vi "RunTest2.vi"(8 "error in (no error)":errorcluster, 11 "Prueba08 in":refnum<class "Prueba08.lvclass">) -> (0 "error out":errorcluster, 2 "resultado":string, 3 "Prueba08 out":refnum<class "Prueba08.lvclass">)   [LabVIEW 2019]
uses:
  <vilib>/Utility/miscctls.llb/LVRowAndColumnTypeDef.ctl
  Prueba/Prueba.lvclass
  Prueba08.lvclass
  Controles/EstadosP08.ctl
  MessageP08.ctl
  Prueba04/Control/Slide.ctl
  Prueba04/Prueba04.lvclass
  QMH/User Event - Stop/User Event - Stop.lvlib
  QMH/Message Queue/Message Queue.lvlib
  QMH/Message Queue/Enqueue Message (Single).vi
  ClusterGEN.ctl
  <vilib>/Utility/error.llb/DialogType.ctl
  <vilib>/Utility/error.llb/Error Cluster From Error Code.vi
  <vilib>/ErrorRing/Error Ring.xnode
  D:/REPO/GitHub/procal/Pruebas/Prueba/Prueba.lvclass
panel:
  out "data":string
  out "fila_tabla":i32
  out "ms":dbl
  out "ms":string[](array[string])
  out "max value":dbl
  out "tablaTipoPondTemp":string[](array[string])
  out "tablaNivelMaxRef":string[](array[string])
  out "Pict Ring 2":u16(ring)
  out "Pict Ring 3":u16(ring)
  out "cumple_no_cumple":bool
  out "Vref":dbl
  in  "Tab":enum32{"Page 1", "Page 2"}(tab)
  out "NivelRMSensayo":dbl=95.0
  out "frecuencia1":dbl=140.0
  out "rangoRef":string
  in  "guardar_Vref":bool
  in  "generar1":bool
  in  "AjusteAmp":T1=50.0 caption="Ajuste de amplitud [mV]" scale=0.0..5000.0
  out "voltaje1":dbl format="%.1f"
  out "frecuencia1":dbl format="%.1f"
  in  "seguir":bool
  in  "guardarParamLEQ":bool caption="PruebaSup"
  in  "Tm":i32=60 min=60
  in  "N":i32=1 min=1 max=9
  in  "TablaTempotal":string[][](table)
  in  "cb_ponderacionTemp":string(combo)="0"
  in  "genera2":bool caption="PruebaSup"
  in  "Tabla":string[][](table)
  in  "salir":bool
  out "cumple":bool
  out "no_cumple":bool
  out "voltaje2":dbl format="%#.1f"
  out "frecuencia2":dbl format="%#.1f"
  # "Elección Señal de Referencia\nsegún marca y modelo de sonómetro"
  # "Nivel RMS para Ensayo"
  # "Rango Referencia"
  # "Frecuencia"
  # "Monitoreo"
  # "Frecuencia"
  # "Hz"
  # "Voltaje"
  # "mV"
  # "8. Respuesta a trenes de ondas. IEC 61672-3: 2006 Cláusula 16"
  # "Tabla Resultados"
  # "Ingrese mediciones\naquí"
  # "Ingrese parámetros"
  # "Seleccione Tone Burst"
  # "N"
  # "Tm"
  # "Solo el máximo valor se \nregistrará en la tabla de Resultados"
  # "Cumple"
  # "No Cumple"
  # "8. Respuesta a trenes de ondas. IEC 61672-3: 2006 Cláusula 16"
  # "Monitoreo"
  # "Nivel RMS para Ensayo"
  # "dB"
  # "Voltaje"
  # "mV"
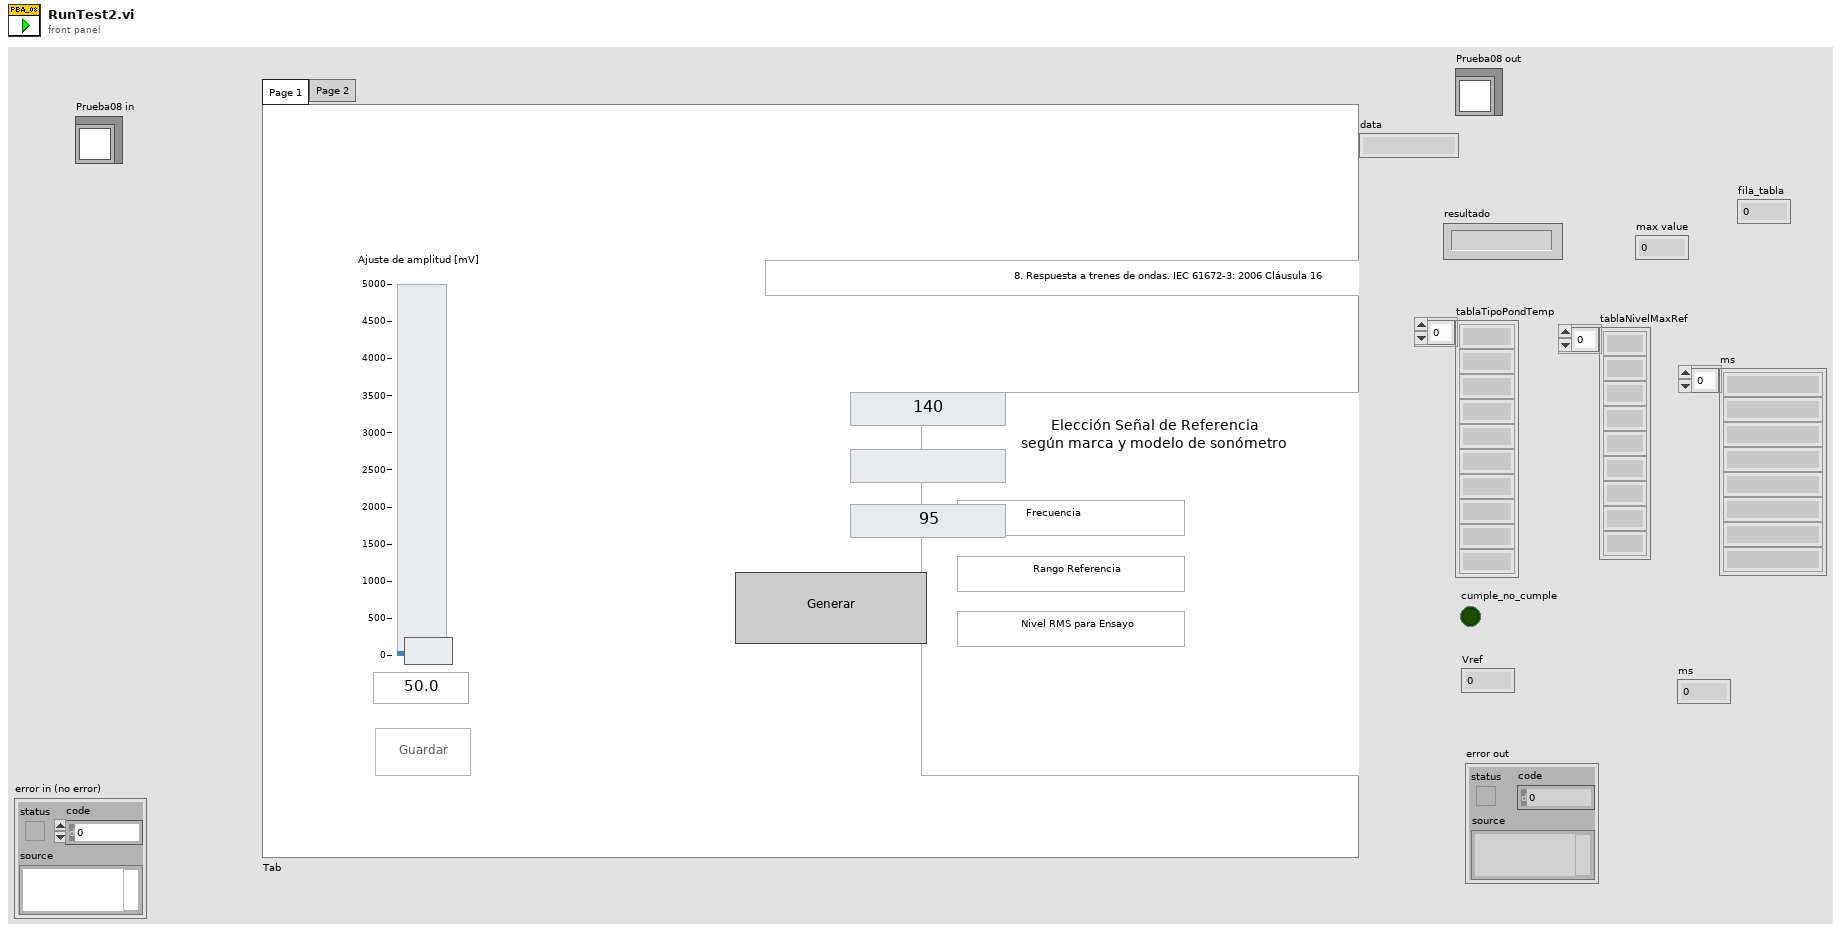
[diagram p1: front panel]
types:
  T1 = typedef "Prueba04.lvclass/Slide.ctl" = dbl
  T2 = typedef "LVRowAndColumnTypeDef.ctl" = cluster{"Row":i32, "Column":i32}
  T3 = typedef "Message Queue.lvlib/All Message Queues.ctl" = cluster{"MHL":refnum<queue>, "Inst_CNT90":refnum<queue>, "Inst_DS360":refnum<queue>, "Inst_Keithley2002":refnum<queue>, "Inst_DAQ":refnum<queue>, "BD":refnum<queue>, "Pistofono":refnum<queue>, "Nexus":refnum<queue>}
  T4 = enum32{"Page 1", "Page 2", "Page 3", "Page 4", "Page 5", "Page 6", "Page 7"}
  T5 = typedef "Prueba08.lvclass/ClusterGEN.ctl" = cluster{"frec":dbl, "amp":dbl, "ms_burst":dbl}
  T6 = enum8{"Enabled", "Disabled", "Disabled and Grayed Out"}
  T7 = cluster{"ControlName":string, "ControlReference":refnum<vi>}[]
  T8 = typedef "Prueba08.lvclass/MessageP08.ctl" = cluster{"Estados":T9, "Data":variant}
  T9 = typedef "Prueba08.lvclass/EstadosP08.ctl" = enum16{"Error", "DetieneInstrumentos", "InicializarInstrumentos", "inicio", "configuraTabla", "FrecAmp1", "FrecAmp2", "nivelMaxRef", "iniciarGEN", "iniciarGEN_burst", "detenerGEN", "llenaTablaTemporal", "guardaVref", "monitoreo", "ingresaMediciones", "guardaMediciones", "cumplimiento", "listo_evaluar", "evaluar", "LeerArchivoConfiguracion", "final", "salir"}
  T10 = typedef "DialogType.ctl" = u16
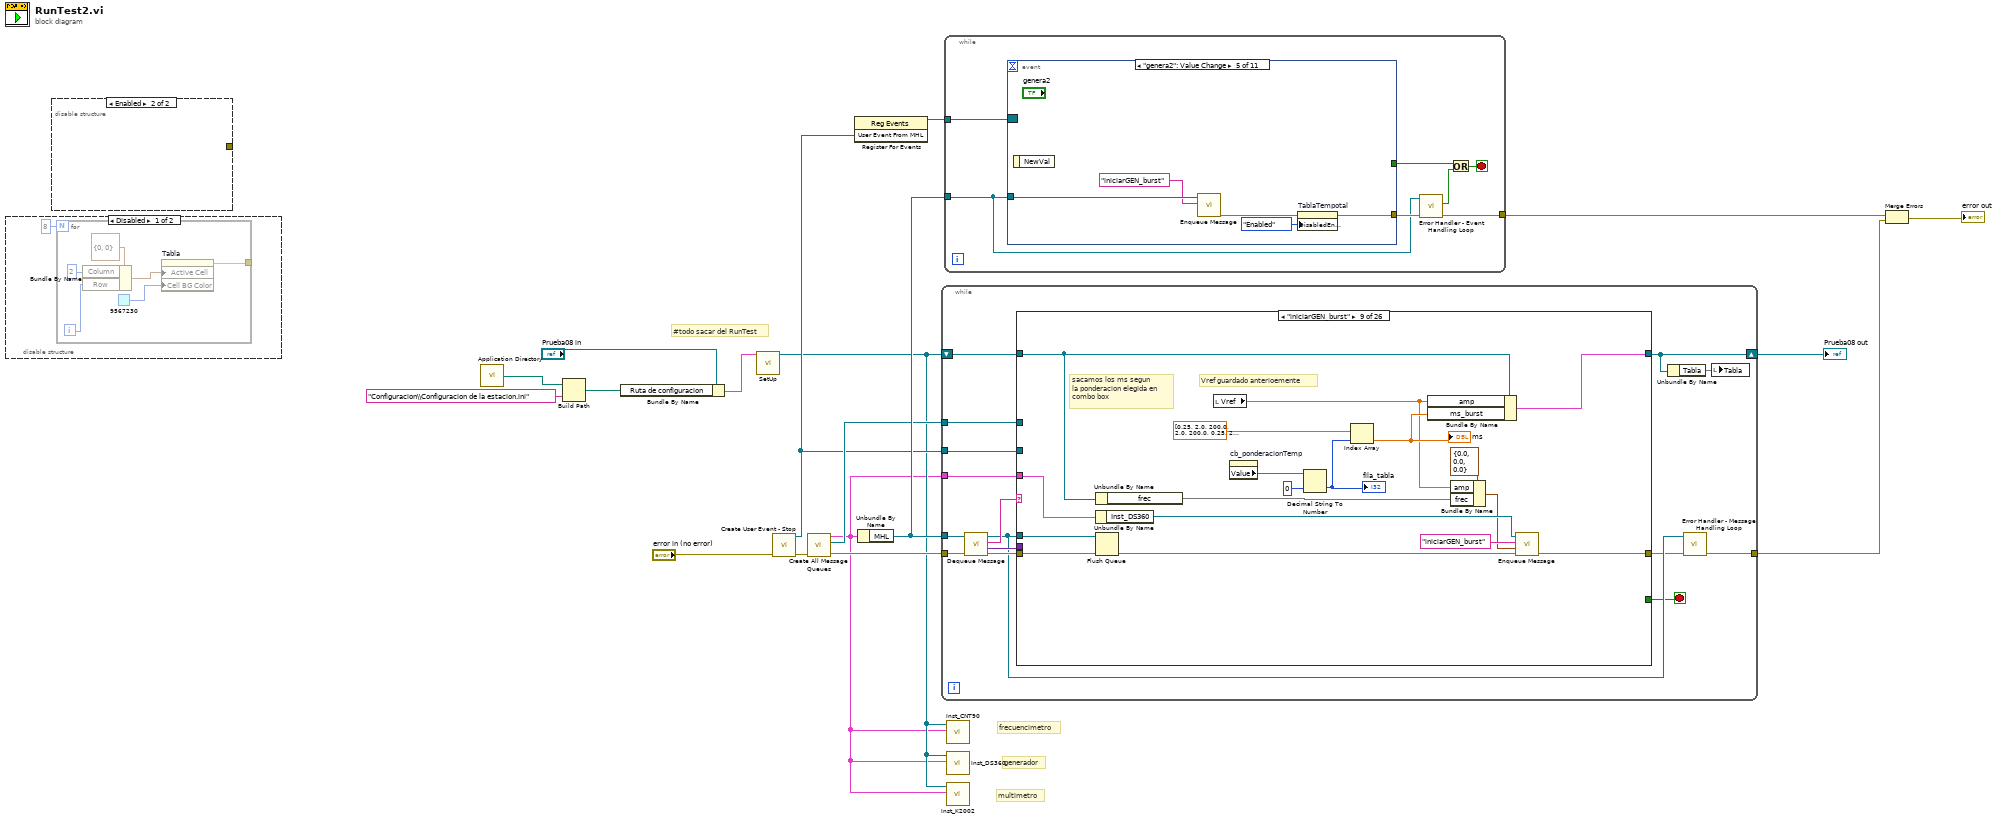
[diagram p0: block diagram]
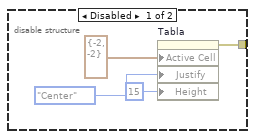
[diagram p3: hidden frame]
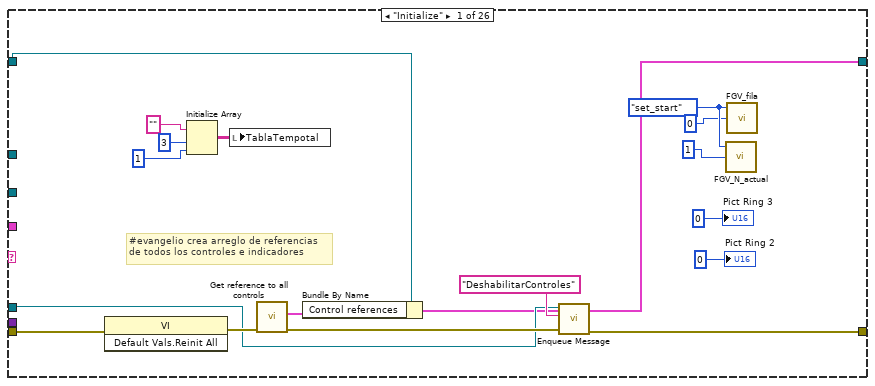
[diagram p4: hidden frame]
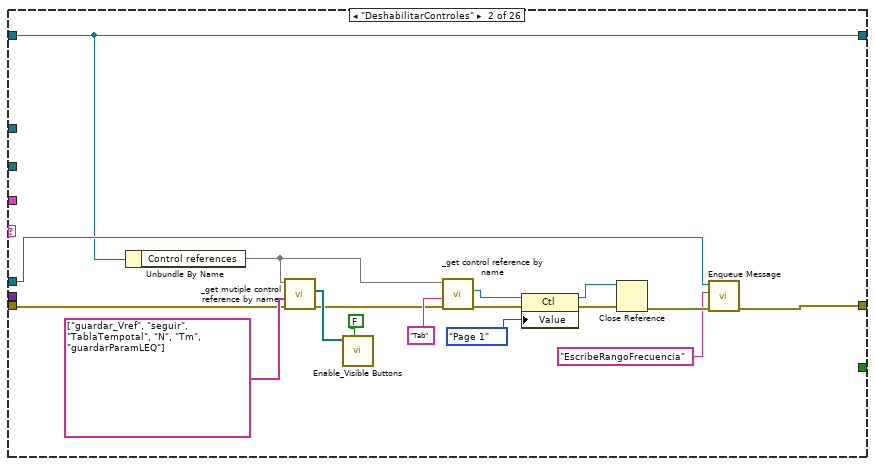
[diagram p5: hidden frame]
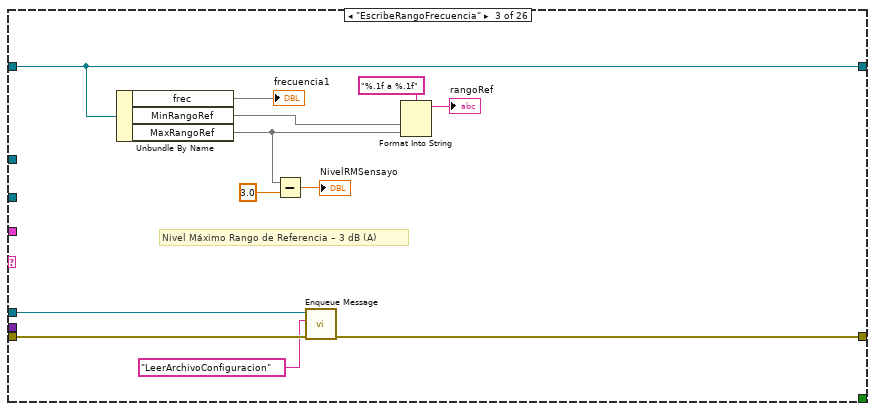
[diagram p6: hidden frame]
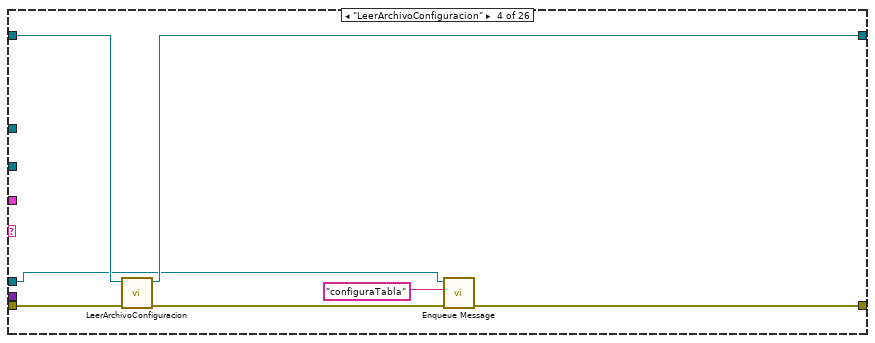
[diagram p7: hidden frame]
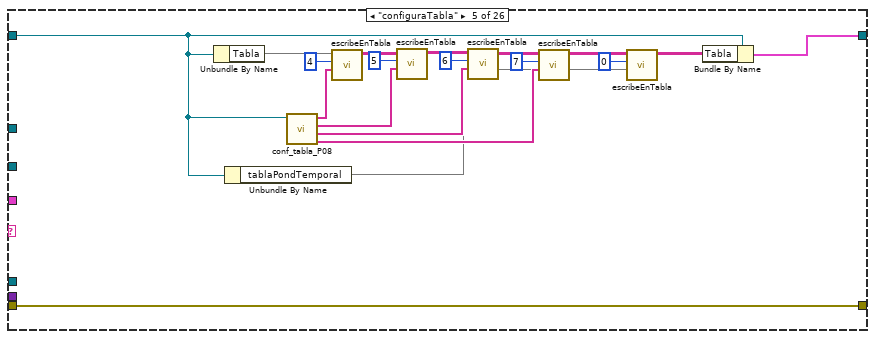
[diagram p8: hidden frame]
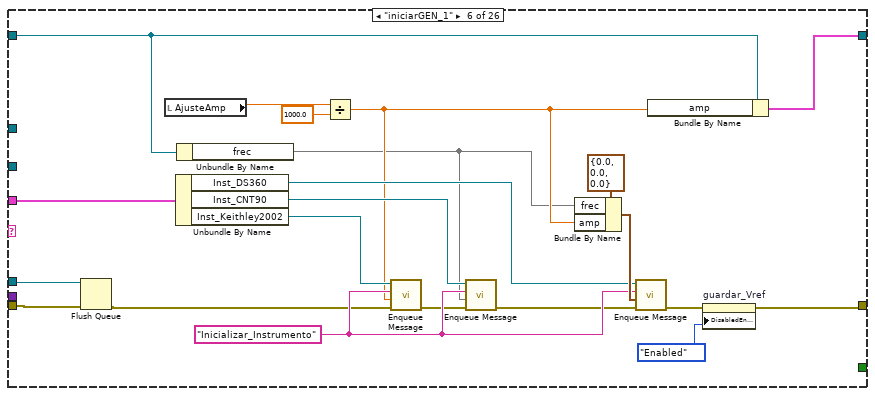
[diagram p9: hidden frame]
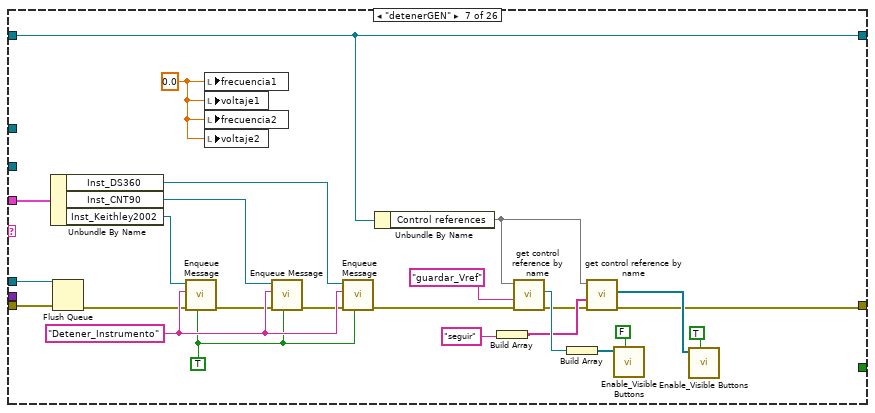
[diagram p10: hidden frame]
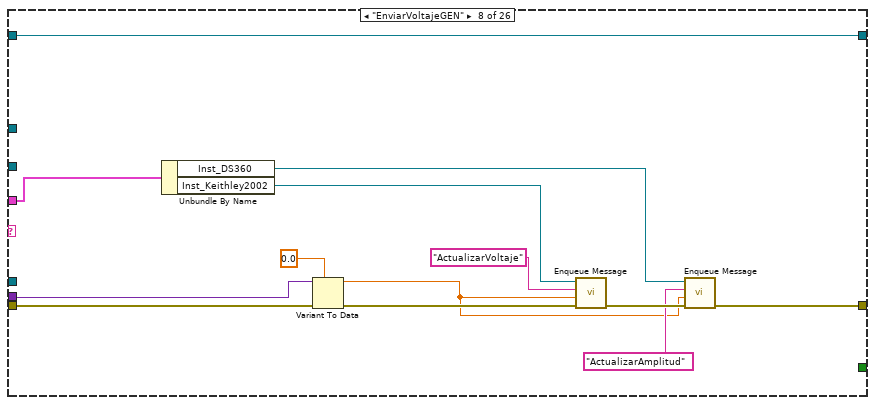
[diagram p11: hidden frame]
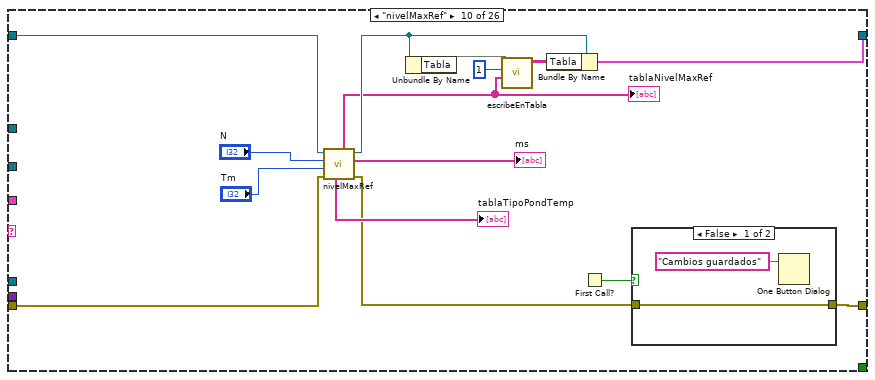
[diagram p12: hidden frame]
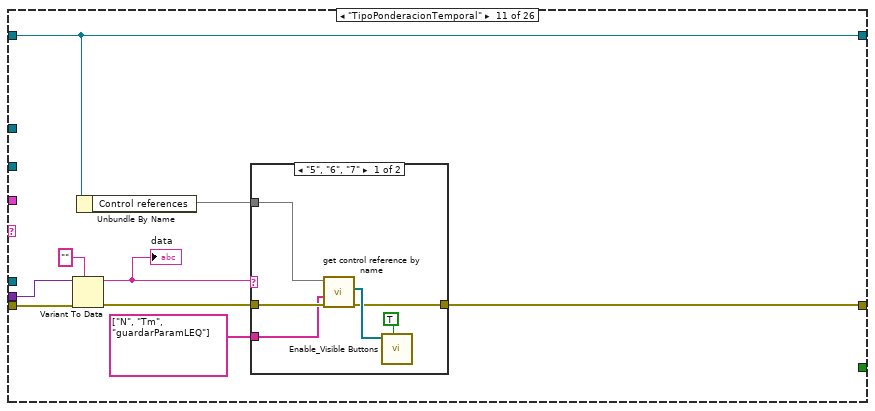
[diagram p14: hidden frame]
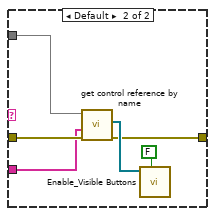
[diagram p15: hidden frame]
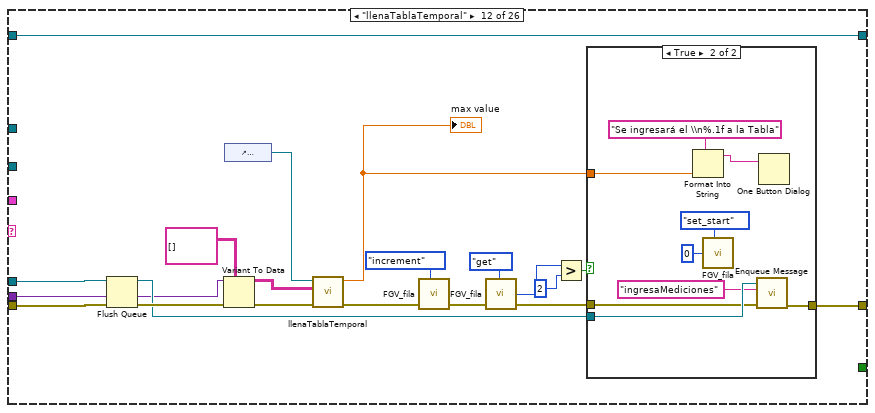
[diagram p16: hidden frame]
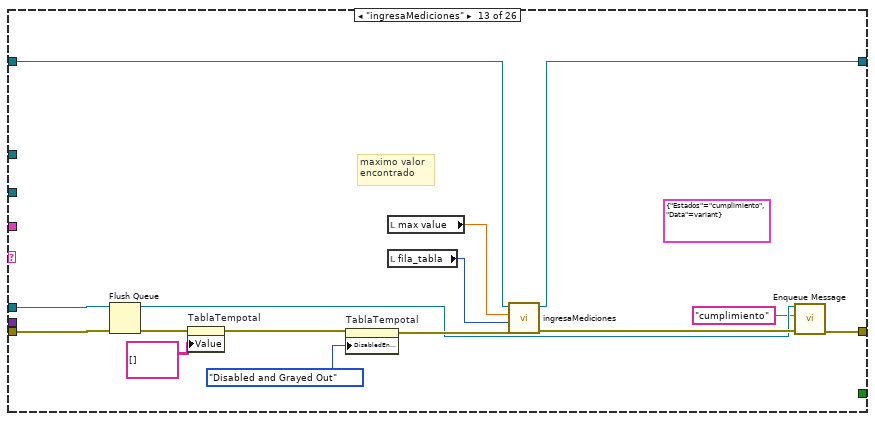
[diagram p18: hidden frame]
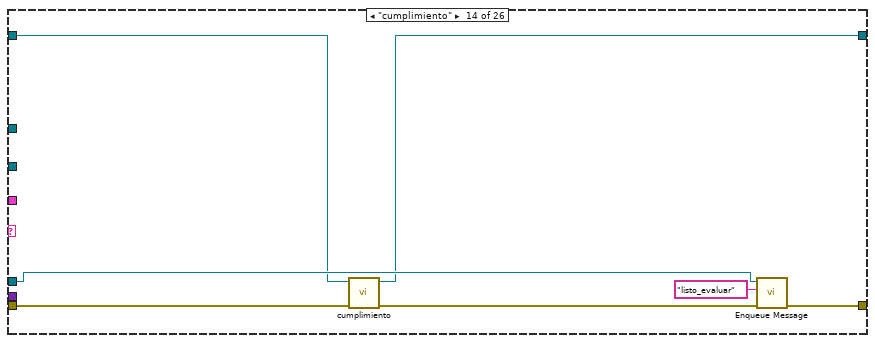
[diagram p19: hidden frame]
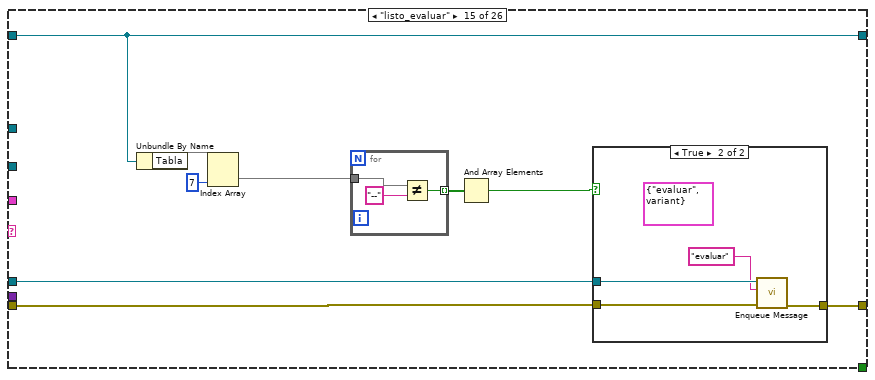
[diagram p20: hidden frame]
diagram:
  # "multimetro"
  # "generador"
  # "frecuencimetro"
  # "#todo sacar del RunTest"
  n1 = disable-structure shown="Disabled" {
    frame Disabled {
      n2 = for {
        N: 8 -> [_]
        tunnel: [w21] -> _
        i -> [w20]
        n3 = Bundle By Name(cluster=T2 {"Row"=0, "Column"=0} ("Active Cell:Active Cell"), "Column"=2, "Row"=w20) -> (w23:T2)
        n4 = property on="Tabla" class="Tbl (strict)"("Active Cell"=w23, "Cell BG Color"=u32 9567230) -> (error out=w21:errorcluster)  [unwired: 2 in, 1 out]
      }
    }
    frame Enabled {
    }
  }
  n5 = disable-structure shown="Enabled" {
    disable-tunnel: [w28 _] -> _
    frame Disabled {
      n6 = property on="Tabla" class="Tbl (strict)"("Active Cell"=T2 {"Row"=-2, "Column"=-2} ("Active Cell:Active Cell"), "Justify"=enum16{"Left", "Center", "Right"}."Center" ("Active Cell:Cell Justification"), "Height"=u32 15 ("Active Cell:Cell Font:Size")) -> (error out=w28:errorcluster)  [unwired: 2 in, 1 out]
    }
    frame Enabled {
    }
  }
  n7 = call <vilib>:"Application Directory.vi"() -> ("Application Directory"=w11:path)
  n8 = Build Path(base path=w11, name or relative path="Configuracion\\Configuracion de la estacion.ini") -> (appended path=w10:path)
  n9 = Bundle By Name(cluster="Prueba08 in", "Ruta de configuracion"=w10) -> (w13:cluster{})
  n10 = call-dynamic "SetUp.vi"("Prueba08 in"=w13) -> ("Prueba08 out"=w2:refnum<class "Prueba08.lvclass">)  [unwired: 9 in, 1 out]
  n11 = call "Create User Event - Stop.vi"("error in (no error)"="error in (no error)") -> ("error out"=w9:errorcluster, "User Event From MHL"=w4:refnum<user-event>)  [unwired: 9 in]
  n12 = call "Create All Message Queues.vi"("error in (no error)"=w9) -> ("error out"=w6:errorcluster, "PL Queues Array"=w5:refnum<queue>[], "All Message Queues out"=w1:T3)  [unwired: 8 in]
  n13 = register-events(w4) -> (reference out=w3:refnum<event-registration>)  [unwired: 2 in, 1 out]
  n14 = Unbundle By Name(w1) -> ("MHL"=w7:refnum<queue>)
  n15 = while {
    tunnel: w7 -> [w41]
    tunnel: w6 -> [w40]
    tunnel: [w34] -> w17
    shift-right: [w42] -> w15
    shift-left: w2 -> [w43]
    tunnel: w1 -> [w33]
    tunnel: w5 -> [w32]
    tunnel: w4 -> [w31]
    stop <- w30 stop-if-true
    n16 = call "Dequeue Message.vi"("error in (no error)"=w40, "Message Queue"=w41) -> ("error out"=w39:errorcluster, "Message Data"=w38:variant, "Message"=w37:string, "dup Message Queue"=w36:refnum<queue>)  [unwired: 6 in]
    n17 = case shown="\"iniciarGEN_burst\"" w37 {
      selector: w37 -> [_ _ _ _ _ _ _ _ _ _ _ _ _ _ _ _ _ _ _ _ _ _ w393 _ w420 _]
      tunnel: w38 -> [_ _ _ _ _ _ _ w164 _ _ w218 w244 _ _ _ _ _ _ w357 w368 _ w387 _ _ _ _]
      tunnel: w39 -> [w58 w66 w83 w98 w111 w125 w143 w165 w192 w206 w219 w251 w266 w283 w292 w308 w314 w321 w360 w371 w376 w388 w397 w408 _ w429]
      tunnel: [w56 w63 w80 w92 w111 w120 w141 w162 w177 w194 w212 w250 w267 w281 w291 w306 w314 w327 w354 w366 w376 w382 w390 w406 w419 w429] -> w35
      tunnel: w36 -> [w57 w65 w82 w94 _ w124 w142 _ w191 _ _ w248 w264 w280 w290 w307 _ w328 _ _ _ w381 w396 w407 _ _]
      tunnel: [w47 w64 w91 w97 w108 w138 w140 w174 w190 w201 w215 w245 w275 w279 w287 w304 w315 w330 w358 w369 w375 w389 w392 w413 w421 w430] -> w42
      tunnel: w43 -> [w48 w64 w91 w96 w100 w119 w140 w174 w176 w207 w215 w245 w276 w278 w287 w304 w315 w330 w359 w370 w375 w389 w392 w413 w421 w430]
      tunnel: w33 -> [_ _ _ _ _ w123 w144 w163 w184 _ _ _ _ _ _ _ _ _ _ _ _ _ _ _ _ _]
      tunnel: w32 -> [_ _ _ _ _ _ _ _ _ _ _ _ _ _ _ _ _ _ _ _ _ _ w395 _ _ _]
      tunnel: w31 -> [_ _ _ _ _ _ _ _ _ _ _ _ _ _ _ _ _ _ _ _ _ _ w394 _ _ _]
      tunnel: [_ _ _ _ _ _ _ _ _ _ _ _ _ _ _ _ _ _ _ _ _ _ w391 _ _ _] -> w30
      frame "Initialize" {
        w50 = enum16{"increment", "set_start", "get"}."set_start" ("action")
        # "#evangelio crea arreglo de referencias\nde todos los controles e indicadores"
        n18 = invoke class="VI" method="Default Vals.Reinit All"(error in=w58) -> (error out=w61:errorcluster)  [unwired: 2 in, 2 out]
        n19 = Initialize Array("", 3 ("dimension size"), 1 ("dimension size")) -> (w55:string[][])
        n20 = local write "TablaTempotal"(w55) -> ()
        n21 = call "Get reference to all controls.vi"("error in (no error)"=w61) -> ("error out"=w59:errorcluster, "Control references"=w60:T7)  [unwired: 5 in]
        n22 = Bundle By Name(cluster=w48, "Control references"=w60) -> (w47:cluster{})
        n23 = call-poly "Enqueue Message.vi"("error in (no error)"=w59, "Message"="DeshabilitarControles", "Message Queue"=w57) -> ("error out"=w56:errorcluster)  [unwired: 7 in, 1 out]
        n24 = call "FGV_N_actual.vi"("N_actual in"=1 ("fila_inicial"), "action"=w50) -> ()  [unwired: 2 in, 2 out]
        n25 = call "FGV_fila.vi"("fila_inicial"=0, "action"=w50) -> ()  [unwired: 2 in, 2 out]
        "Pict Ring 2" <- u16 0 ("Pict Ring 2")
        "Pict Ring 3" <- u16 0 ("Pict Ring 3")
      }
      frame "DeshabilitarControles" {
        n26 = Unbundle By Name(w64) -> ("Control references"=w75)
        n27 = call "_get mutiple control reference by name.vi"("error in (no error)"=w66, "Control names"=string[] ["guardar_Vref", "seguir", "TablaTempotal", "N", "Tm", "guardarParamLEQ"], "Control references"=w75) -> ("error out"=w72:errorcluster, "References"=w73:refnum<vi>[])  [unwired: 3 in]
        n28 = call "Enable_Visible Buttons.vi"("Enable? (T)"=FALSE, "Controls Ref Array"=w73) -> ()  [unwired: 10 in]
        n29 = call "_get control reference by name.vi"("error in (no error)"=w72, "Control name"="Tab" ("Message"), "Control references"=w75) -> ("error out"=w79:errorcluster, "Ctl Refnum"=w77:refnum<vi>)  [unwired: 3 in]
        n30 = property class="Ctl"(reference=w77, error in=w79, "Value"=T4."Page 1" ("Tab_Prueba04")) -> (reference out=w68:refnum<vi>, error out=w70:errorcluster)
        n31 = Close Reference(reference=w68, error in (no error)=w70) -> (error out=w69:errorcluster)
        n32 = call-poly "Enqueue Message.vi"("error in (no error)"=w69, "Message"="EscribeRangoFrecuencia", "Message Queue"=w65) -> ("error out"=w63:errorcluster)  [unwired: 7 in, 1 out]
      }
      frame "EscribeRangoFrecuencia" {
        # "Nivel Máximo Rango de Referencia – 3 dB (A)"
        n33 = Unbundle By Name(w91) -> ("frec"=→"frecuencia1", "MinRangoRef"=w87, "MaxRangoRef"=w86)
        n34 = Subtract(x=w86, y=3.0) -> (x-y=→"NivelRMSensayo":dbl)
        n35 = call-poly "Enqueue Message.vi"("error in (no error)"=w83, "Message"="LeerArchivoConfiguracion", "Message Queue"=w82) -> ("error out"=w80:errorcluster)  [unwired: 7 in, 1 out]
        n36 = Format Into String(format string="%.1f a %.1f", w87, w86) -> (resulting string=→"rangoRef":string)  [unwired: 2 in, 1 out]
      }
      frame "LeerArchivoConfiguracion" {
        n37 = call "LeerArchivoConfiguracion.vi"("error in"=w98, "Prueba31 in"=w96) -> ("error out"=w95:errorcluster, "Prueba31 out"=w97:refnum<class "Prueba08.lvclass">)  [unwired: 8 in]
        n38 = call-poly "Enqueue Message.vi"("error in (no error)"=w95, "Message"="configuraTabla", "Message Queue"=w94) -> ("error out"=w92:errorcluster)  [unwired: 7 in, 1 out]
      }
      frame "configuraTabla" {
        n39 = Unbundle By Name(w100) -> ("Tabla"=w107)
        n40 = Unbundle By Name(w100) -> ("tablaPondTemporal"=w99)
        n41 = call "conf_tabla_P08.vi"("Prueba07 out"=w100) -> ("cumplimiento"=w103:string[], "Tol -"=w104:string[], "Tol +"=w105:string[], "incertidumbre"=w106:string[])  [unwired: 7 in]
        n42 = call "escribeEnTabla.vi"("parametros"=w106, "col"=4, "tabla in"=w107) -> ("tabla out"=w117:string[][])  [unwired: 8 in]
        n43 = call "escribeEnTabla.vi"("parametros"=w105, "col"=5, "tabla in"=w117) -> ("tabla out"=w116:string[][])  [unwired: 8 in]
        n44 = call "escribeEnTabla.vi"("parametros"=w104, "col"=6, "tabla in"=w116) -> ("tabla out"=w112:string[][])  [unwired: 8 in]
        n45 = call "escribeEnTabla.vi"("parametros"=w103, "col"=7, "tabla in"=w112) -> ("tabla out"=w110:string[][])  [unwired: 8 in]
        n46 = call "escribeEnTabla.vi"("parametros"=w99, "col"=0, "tabla in"=w110) -> ("tabla out"=w102:string[][])  [unwired: 8 in]
        n47 = Bundle By Name(cluster=w100, "Tabla"=w102) -> (w108:cluster{})
      }
      frame "iniciarGEN_1" {
        w133 = "Inicializar_Instrumento" ("Message")
        n48 = Flush Queue(queue=w124, error in (no error)=w125) -> (error out=w127:errorcluster)  [unwired: 2 out]
        n49 = local read "AjusteAmp"() -> (w137:T1)
        n50 = Unbundle By Name(w123) -> ("Inst_DS360"=w128:refnum<queue>, "Inst_CNT90"=w126:refnum<queue>, "Inst_Keithley2002"=w135:refnum<queue>)
        n51 = Unbundle By Name(w119) -> ("frec"=w118)
        n52 = Divide(x=w137, y=T1 1000.0) -> (x/y=w121:T1)
        n53 = call-poly "Enqueue Message.vi"("error in (no error)"=w127, "Message Data"=w121, "Message"=w133, "Message Queue"=w135) -> ("error out"=w132:errorcluster)  [unwired: 6 in, 1 out]
        n54 = call-poly "Enqueue Message.vi"("error in (no error)"=w132, "Message Data"=w118, "Message"=w133, "Message Queue"=w126) -> ("error out"=w131:errorcluster)  [unwired: 6 in, 1 out]
        n55 = Bundle By Name(cluster=T5 {"frec"=0.0, "amp"=0.0, "ms_burst"=0.0} ("clusterGEN"), "frec"=w118, "amp"=w121) -> (w134:T5)
        n56 = call-poly "Enqueue Message.vi"("error in (no error)"=w131, "Message Data"=w134, "Message"=w133, "Message Queue"=w128) -> ("error out"=w129:errorcluster)  [unwired: 6 in, 1 out]
        n57 = Bundle By Name(cluster=w119, "amp"=w121) -> (w138:cluster{})
        n58 = property on="guardar_Vref" class="Bool"(error in=w129, "DisabledEnum"=T6."Enabled" ("Disabled")) -> (error out=w120:errorcluster)  [unwired: 1 in, 1 out]
      }
      frame "detenerGEN" {
        w139 = 0.0 ("frecuencia1")
        w157 = TRUE ("Priority Message? (F)")
        w158 = "Detener_Instrumento"
        n59 = Unbundle By Name(w144) -> ("Inst_DS360"=w159:refnum<queue>, "Inst_CNT90"=w160:refnum<queue>, "Inst_Keithley2002"=w161:refnum<queue>)
        n60 = Flush Queue(queue=w142, error in (no error)=w143) -> (error out=w146:errorcluster)  [unwired: 2 out]
        n61 = call-poly "Enqueue Message.vi"("Priority Message? (F)"=w157, "Message"=w158, "Message Queue"=w161) -> ()  [unwired: 7 in, 2 out]
        n62 = local write "frecuencia1"(w139) -> ()
        n63 = local write "voltaje1"(w139) -> ()
        n64 = local write "frecuencia2"(w139) -> ()
        n65 = local write "voltaje2"(w139) -> ()
        n66 = call-poly "Enqueue Message.vi"("Priority Message? (F)"=w157, "Message"=w158, "Message Queue"=w160) -> ()  [unwired: 7 in, 2 out]
        n67 = call-poly "Enqueue Message.vi"("Priority Message? (F)"=w157, "error in (no error)"=w146, "Message"=w158, "Message Queue"=w159) -> ("error out"=w155:errorcluster)  [unwired: 6 in, 1 out]
        n68 = Unbundle By Name(w140) -> ("Control references"=w150)
        n69 = Build Array("seguir" ("String")) -> (w147:string[])
        n70 = call-poly "get control reference by name.vi"("error in (no error)"=w155, "Control name"="guardar_Vref" ("String"), "Control references"=w150) -> ("error out"=w145:errorcluster, "Ctl Refnum"=w153:refnum<vi>)  [unwired: 3 in]
        n71 = Build Array(w153) -> (w152:refnum<vi>[])
        n72 = call-poly "get control reference by name.vi"("error in (no error)"=w145, "Control names"=w147, "Control references"=w150) -> ("error out"=w141:errorcluster, "References"=w149:refnum<vi>[])  [unwired: 3 in]
        n73 = call "Enable_Visible Buttons.vi"("Enable? (T)"=FALSE, "Controls Ref Array"=w152) -> ()  [unwired: 10 in]
        n74 = call "Enable_Visible Buttons.vi"("Enable? (T)"=TRUE, "Controls Ref Array"=w149) -> ()  [unwired: 10 in]
      }
      frame "EnviarVoltajeGEN" {
        n75 = Unbundle By Name(w163) -> ("Inst_DS360"=w168:refnum<queue>, "Inst_Keithley2002"=w173:refnum<queue>)
        n76 = Variant To Data(error in=w165, type=0.0, Variant=w164) -> (data=w166:dbl, error out=w171:errorcluster)
        n77 = call-poly "Enqueue Message.vi"("error in (no error)"=w171, "Message Data"=w166, "Message"="ActualizarVoltaje", "Message Queue"=w173) -> ("error out"=w169:errorcluster)  [unwired: 6 in, 1 out]
        n78 = call-poly "Enqueue Message.vi"("error in (no error)"=w169, "Message Data"=w166, "Message"="ActualizarAmplitud", "Message Queue"=w168) -> ("error out"=w162:errorcluster)  [unwired: 6 in, 1 out]
      }
      frame "iniciarGEN_burst" {
        # "sacamos los ms segun\nla ponderacion elegida en\ncombo box"
        # "Vref guardado anterioemente"
        n79 = Unbundle By Name(w184) -> ("Inst_DS360"=w182:refnum<queue>)
        n80 = Flush Queue(queue=w191, error in (no error)=w192) -> (error out=w183:errorcluster)  [unwired: 2 out]
        n81 = Unbundle By Name(w176) -> ("frec"=w175)
        n82 = local read "Vref"() -> (w178:dbl)
        n83 = property on="cb_ponderacionTemp" class="CmbBox"() -> ("Value"=w187:string)  [unwired: 2 in, 2 out]
        n84 = Decimal String To Number(string=w187, default (0L)=0 ("default (0 I32)")) -> (number=w185:i32)  [unwired: 1 in, 1 out]
        "fila_tabla" <- w185
        n85 = Index Array(array=dbl[] [0.25, 2.0, 200.0, 2.0, 200.0, 0.25, 2.0, 200.0], index=w185) -> (element=w188:dbl)
        "ms" <- w188
        n86 = Bundle By Name(cluster=w176, "amp"=w178, "ms_burst"=w188) -> (w190:cluster{})
        n87 = Bundle By Name(cluster=T5 {"frec"=0.0, "amp"=0.0, "ms_burst"=0.0} ("clusterGEN"), "amp"=w178, "frec"=w175) -> (w179:T5)
        n88 = call-poly "Enqueue Message.vi"("error in (no error)"=w183, "Message Data"=w179, "Message"="iniciarGEN_burst", "Message Queue"=w182) -> ("error out"=w177:errorcluster)  [unwired: 6 in, 1 out]
      }
      frame "nivelMaxRef" {
        n89 = call "nivelMaxRef.vi"("error in (no error)"=w206, "Tm"="Tm", "N"="N", "Prueba08 in"=w207) -> ("error out"=w195:errorcluster, "ms"=→"ms":string[], "Prueba08 out"=w205:refnum<class "Prueba08.lvclass">, "tablaNivelMaxRef"=w202:string[], "tablaTipoPondTemp"=→"tablaTipoPondTemp":string[])  [unwired: 2 in, 1 out]
        "tablaNivelMaxRef" <- w202
        n90 = Unbundle By Name(w205) -> ("Tabla"=w204)
        n91 = call "escribeEnTabla.vi"("parametros"=w202, "col"=1, "tabla in"=w204) -> ("tabla out"=w200:string[][])  [unwired: 8 in]
        n92 = Bundle By Name(cluster=w205, "Tabla"=w200) -> (w201:cluster{})
        n93 = First Call?() -> (First Call?: T/F=w193:bool)
        n94 = case shown="False" w193 {
          tunnel: w195 -> [w208 w210]
          tunnel: [w208 w210] -> w194
          frame False {
            n95 = One Button Dialog(message="Cambios guardados") -> ()  [unwired: 1 in, 1 out]
          }
          frame True {
          }
        }
      }
      frame "TipoPonderacionTemporal" {
        n96 = Variant To Data(error in=w219, type="", Variant=w218) -> (data=w216:string, error out=w213:errorcluster)
        "data" <- w216
        n97 = Unbundle By Name(w215) -> ("Control references"=w214)
        n98 = case shown="\"5\", \"6\", \"7\"" w216 {
          tunnel: w214 -> [w222 w228]
          tunnel: w213 -> [w221 w227]
          tunnel: [w223 w229] -> w212
          tunnel: string[] ["N", "Tm", "guardarParamLEQ"] ("String") -> [w220 w226]
          frame "5", "6", "7" {
            n99 = call-poly "get control reference by name.vi"("error in (no error)"=w221, "Control names"=w220, "Control references"=w222) -> ("error out"=w223:errorcluster, "References"=w224:refnum<vi>[])  [unwired: 3 in]
            n100 = call "Enable_Visible Buttons.vi"("Enable? (T)"=TRUE, "Controls Ref Array"=w224) -> ()  [unwired: 10 in]
          }
          frame Default {
            n101 = call-poly "get control reference by name.vi"("error in (no error)"=w227, "Control names"=w226, "Control references"=w228) -> ("error out"=w229:errorcluster, "References"=w230:refnum<vi>[])  [unwired: 3 in]
            n102 = call "Enable_Visible Buttons.vi"("Enable? (T)"=FALSE, "Controls Ref Array"=w230) -> ()  [unwired: 10 in]
          }
        }
      }
      frame "llenaTablaTemporal" {
        n103 = Flush Queue(queue=w248, error in (no error)=w251) -> (queue out=w247:refnum<queue>, error out=w249:errorcluster)  [unwired: 1 out]
        n104 = Variant To Data(error in=w249, type=string[][] [] ("NewVal"), Variant=w244) -> (data=w242:string[][], error out=w241:errorcluster)
        n105 = control-ref of="TablaTempotal"() -> (w243:refnum<vi>)
        n106 = call "llenaTablaTemporal.vi"("Tbl Refnum"=w243, "New Value"=w242, "error out"=w241) -> ("max value"=w232:dbl, "error in (no error)"=w240:errorcluster)  [unwired: 6 in]
        "max value" <- w232
        n107 = call "FGV_fila.vi"("error in (no error)"=w240, "action"=enum16{"increment", "set_start", "get"}."increment") -> ("error out"=w239:errorcluster)  [unwired: 2 in, 1 out]
        n108 = call "FGV_fila.vi"("error in (no error)"=w239, "action"=enum16{"increment", "set_start", "get"}."get") -> ("error out"=w237:errorcluster, "fila out"=w235:i32)  [unwired: 2 in]
        n109 = Greater?(x=w235, y=2) -> (0:w233:bool)
        n110 = case shown="True" w233 {
          tunnel: [w252 w261] -> w250
          tunnel: w247 -> [_ w260]
          tunnel: w237 -> [w252 w259]
          tunnel: w232 -> [_ w255]
          frame False {
          }
          frame True {
            n111 = Format Into String(format string="Se ingresará el \\n%.1f a la Tabla" ("message"), w255) -> (resulting string=w254:string)  [unwired: 2 in, 1 out]
            n112 = call "FGV_fila.vi"("fila_inicial"=0, "action"=enum16{"increment", "set_start", "get"}."set_start") -> ()  [unwired: 2 in, 2 out]
            n113 = call-poly "Enqueue Message.vi"("error in (no error)"=w259, "Message"="ingresaMediciones", "Message Queue"=w260) -> ("error out"=w261:errorcluster)  [unwired: 7 in, 1 out]
            n114 = One Button Dialog(message=w254) -> ()  [unwired: 1 in, 1 out]
          }
        }
      }
      frame "ingresaMediciones" {
        (unwired) T8 {"Estados"=enum."cumplimiento", "Data"=variant} ("element")
        # "maximo valor\nencontrado"
        n115 = Flush Queue(queue=w264, error in (no error)=w266) -> (queue out=w263:refnum<queue>, error out=w265:errorcluster)  [unwired: 1 out]
        n116 = property on="TablaTempotal" class="Tbl (strict)"(error in=w265, "Value"=string[][] [] ("TablaTempotal")) -> (error out=w271:errorcluster)  [unwired: 1 in, 1 out]
        n117 = property on="TablaTempotal" class="Tbl (strict)"(error in=w271, "DisabledEnum"=T6."Disabled and Grayed Out" ("Disabled")) -> (error out=w270:errorcluster)  [unwired: 1 in, 1 out]
        n118 = local read "max value"() -> (w274:dbl)
        n119 = local read "fila_tabla"() -> (w273:i32)
        n120 = call "ingresaMediciones.vi"("error in (no error)"=w270, "fila tabla"=w273, "max value"=w274, "Prueba08 in"=w276) -> ("error out"=w268:errorcluster, "Prueba08 out"=w275:refnum<class "Prueba08.lvclass">)  [unwired: 6 in]
        n121 = call-poly "Enqueue Message.vi"("error in (no error)"=w268, "Message"="cumplimiento", "Message Queue"=w263) -> ("error out"=w267:errorcluster)  [unwired: 7 in, 1 out]
      }
      frame "cumplimiento" {
        n122 = call "cumplimiento.vi"("error in (no error)"=w283, "Prueba08 in"=w278) -> ("error out"=w282:errorcluster, "Prueba08 out"=w279:refnum<class "Prueba08.lvclass">)  [unwired: 8 in]
        n123 = call-poly "Enqueue Message.vi"("error in (no error)"=w282, "Message"="listo_evaluar", "Message Queue"=w280) -> ("error out"=w281:errorcluster)  [unwired: 7 in, 1 out]
      }
      frame "listo_evaluar" {
        n124 = Unbundle By Name(w287) -> ("Tabla"=w286)
        n125 = Index Array(array=w286, index (col)=7 ("disabled index (col)")) -> (element=w285)  [unwired: 1 in]
        n126 = for {
          tunnel: [w300] -> w288 mode=indexing
          tunnel: w285 -> [w298]
          n127 = Not Equal?(x=w298, y="--") -> (x != y?=w300:bool)
        }
        n128 = And Array Elements(Boolean array=w288) -> (logical AND=w284:bool)
        n129 = case shown="True" w284 {
          tunnel: w292 -> [w293 w297]
          tunnel: [w293 w296] -> w291
          tunnel: w290 -> [_ w295]
          frame False {
          }
          frame True {
            (unwired) T8 {"Estados"=enum."evaluar", "Data"=variant} ("MessageP08")
            n130 = call-poly "Enqueue Message.vi"("error in (no error)"=w297, "Message"="evaluar", "Message Queue"=w295) -> ("error out"=w296:errorcluster)  [unwired: 7 in, 1 out]
          }
        }
      }
      frame "evaluar" {
        # "si todos cumplen\nentonces el ensayo\ncumple"
        n131 = Unbundle By Name(w304) -> ("Tabla"=w303)
        n132 = call-poly "Enqueue Message.vi"("error in (no error)"=w308, "Message"="final", "Message Queue"=w307) -> ("error out"=w306:errorcluster)  [unwired: 7 in, 1 out]
        n133 = Index Array(array=w303, index (col)=7 ("disabled index (col)")) -> (element=w302)  [unwired: 1 in]
        n134 = for {
          tunnel: [w313] -> w310 mode=indexing
          tunnel: w302 -> [w311]
          n135 = Equal?(x=w311, y="Cumple") -> (x = y?=w313:bool)
        }
        n136 = And Array Elements(Boolean array=w310) -> (logical AND=→"cumple_no_cumple":bool)
      }
      frame "final" {
        n137 = local read "cumple_no_cumple"() -> (w316:bool)
        "cumple" <- w316
        n138 = Not(x=w316) -> (.not. x?=→"no_cumple":bool)
        n139 = Select(t="Cumple", s=w316, f="No Cumple") -> (s? t:f=→"resultado":string)
      }
      frame "iniciarGEN_burst_2" {
        n140 = property on="cb_ponderacionTemp" class="CmbBox"(error in=w321) -> ("Value"=w324:string)  [unwired: 1 in, 2 out]
        n141 = local read "N"() -> (w326:i32)
        n142 = local read "Tm"() -> (w329:i32)
        n143 = case shown="\"5\"..\"7\"" w324 {
          tunnel: w321 -> [w334 w345]
          tunnel: w329 -> [w333 w344]
          tunnel: w326 -> [_ w343]
          tunnel: [w332 w340] -> w323
          tunnel: [2 ("N_actual out") w339] -> w322
          frame "0".."4", Default {
            n144 = disable-structure shown="Disabled" {
              disable-tunnel: w334 -> [w337 w338]
              disable-tunnel: w333 -> [w336 _]
              disable-tunnel: [w335 w338] -> w332
              frame Disabled {
                n145 = call "estadoToneBurst_FastSlow.vi"("error in (no error)"=w337, "Tm"=w336) -> ("error out"=w335:errorcluster)  [unwired: 9 in]
              }
              frame Enabled {
              }
            }
          }
          frame "5".."7" {
            n146 = call "estadoToneBurst.vi"("error in (no error)"=w345, "Tm"=w344, "N"=w343) -> ("error out"=w341:errorcluster)  [unwired: 7 in, 1 out]
            n147 = call "FGV_N_actual.vi"("error in (no error)"=w341, "action"=enum16{"increment", "set_start", "get"}."increment") -> ("error out"=w340:errorcluster, "N_actual out"=w339:i32)  [unwired: 2 in]
          }
        }
        n148 = Greater?(x=w322, y=w326) -> (0:w325:bool)
        n149 = case shown="True" w325 {
          tunnel: w328 -> [w349 _]
          tunnel: [w348 w353] -> w327
          tunnel: w323 -> [w347 w353]
          frame False {
            n150 = call-poly "Enqueue Message.vi"("error in (no error)"=w347, "Message"="iniciarGEN_burst", "Message Queue"=w349) -> ("error out"=w348:errorcluster)  [unwired: 7 in, 1 out]
          }
          frame True {
            n151 = One Button Dialog(message="Ingrese las mediciones \nen la Tabla Temporal") -> ()  [unwired: 1 in, 1 out]
            n152 = call "FGV_N_actual.vi"("N_actual in"=1, "action"=enum16{"increment", "set_start", "get"}."set_start") -> ()  [unwired: 2 in, 2 out]
          }
        }
      }
      frame "DatoRecibidoCNT90" {
        n153 = Variant To Data(error in=w360, type=0.0 ("y"), Variant=w357) -> (data=w355:dbl, error out=w354:errorcluster)
        "frecuencia2" <- w355
        "frecuencia1" <- w355
        n154 = Bundle By Name(cluster=w359, "frecMedida"=w355) -> (w358:cluster{})
      }
      frame "DatoRecibidoK2002" {
        n155 = Variant To Data(error in=w371, type=0.0 ("y"), Variant=w368) -> (data=w362:dbl, error out=w366:errorcluster)
        n156 = Multiply(x=w362, y=1000.0) -> (x*y=w361:dbl)
        "voltaje2" <- w361
        n157 = Multiply(x=w362, y=1000.0) -> (x*y=→"voltaje1":dbl)
        n158 = Bundle By Name(cluster=w370, "voltMedido"=w361) -> (w369:cluster{})
      }
      frame "guardaVref" {
        n159 = local read "AjusteAmp"() -> (w374:T1)
        n160 = Divide(x=w374, y=T1 1000.0) -> (x/y=w372:T1)
        "Vref" <- w372
        n161 = Number To Fractional String(number=w372, precision (6)=i16 3) -> (F-format string=w377:string)  [unwired: 2 in]
        n162 = Format Into String(format string="Se guardó Vref = %s volts", w377) -> (resulting string=w380:string)  [unwired: 2 in, 1 out]
        n163 = One Button Dialog(message=w380) -> ()  [unwired: 1 in, 1 out]
      }
      frame "Error" {
        w385 = T10 1 items=["no dialog", "OK message", "continue or stop message", "OK message + warnings", "continue/stop + warnings"] ("type of dialog (OK msg:1)")
        n164 = Variant To Data(error in=w388, type=w388, Variant=w387) -> (data=w386:errorcluster, error out=w383:errorcluster)
        n165 = call <vilib>:"Simple Error Handler.vi"("type of dialog (OK msg:1)"=w385, "error in (no error)"=w386) -> ()  [unwired: 3 in, 5 out]
        n166 = call-poly "Enqueue Message.vi"("error in (no error)"=w383, "Message"="Exit", "Message Queue"=w381) -> ("error out"=w382:errorcluster)  [unwired: 7 in, 1 out]
      }
      frame "Exit" {
        w391 = TRUE
        # "#evangelio Manda a cerrar el EHL"
        # "#evangelio Manda a cerrar todos los Loops"
        n167 = Release Queue(queue=w396, error in (no error)=w397) -> (error out=w401:errorcluster)  [unwired: 1 in, 2 out]
        n168 = Unbundle By Name(w392) -> ("Control references"=w402)
        n169 = for {
          tunnel: w395 -> [w405] mode=indexing
          tunnel: w393 -> [w404]
          tunnel: TRUE -> [w403]
          n170 = call-poly "Enqueue Message.vi"("Priority Message? (F)"=w403, "Message"=w404, "Message Queue"=w405) -> ()  [unwired: 7 in, 2 out]
        }
        n171 = call "Close All Ref.vi"("error in (no error)"=w401, "Control references"=w402) -> ("error out"=w399:errorcluster)  [unwired: 9 in]
        n172 = call "Fire User Event - Stop.vi"("error in (no error)"=w399, "Event Data"=w391, "User Event"="Exit EHL", "User Event in"=w394) -> ("error out"=w390:errorcluster)  [unwired: 7 in]
      }
      frame "Confirmar Salida" {
        n173 = Two Button Dialog(message="¿Quieres cerrar la aplicación?", 1:"No" ("T button name (\"OK\")"), 2:"Si" ("T button name (\"OK\")")) -> (T button?=w409:bool)
        n174 = case shown="True" w409 {
          tunnel: w408 -> [w414 w418]
          tunnel: [w414 w417] -> w406
          tunnel: w407 -> [_ w415]
          frame False {
          }
          frame True {
            n175 = call-poly "Enqueue Message.vi"("error in (no error)"=w418, "Message"="Exit", "Message Queue"=w415) -> ("error out"=w417:errorcluster)  [unwired: 7 in, 1 out]
          }
        }
      }
      frame Default {
        n176 = xnode "Error Ring"("parameter 0"=w420) -> ("error out"=w419:errorcluster)
      }
      frame "----------------------Controles----------------------" {
      }
    }
    n177 = Unbundle By Name(w42) -> ("Tabla"=w44)
    n178 = call "Error Handler - Message Handling Loop.vi"("error in (no error)"=w35, "Message Queue"=w36) -> ("dup error in"=w34:errorcluster)  [unwired: 8 in, 1 out]
    n179 = local write "Tabla"(w44) -> ()
  }
  "Prueba08 out" <- w15
  n180 = while {
    tunnel: w7 -> [w431]
    tunnel: [w433] -> w18
    tunnel: w3 -> [w436]
    stop <- w437 stop-if-true
    n181 = event shown="[4] \"genera2\": Value Change" {
      selector: w436 -> [_ _ _ _ _ _ _ _ _ _ _]
      dyn-events: _ -> [_ _ _ _ _ _ _ _ _ _ _]
      timeout: _ -> [_ _ _ _ _ _ _ _ _ _ _]
      tunnel: w431 -> [w440 _ w448 w454 w460 w465 w467 w473 w479 w483 w487]
      tunnel: [w439 _ _ w455 w456 w462 w468 w474 w476 w482 w484] -> w434
      tunnel: [_ w441 _ _ _ _ _ _ _ _ _] -> w435
      event "salir": Value Change {
        n182 = event-data() -> ()  [unwired: 1 in, 1 out]
        n183 = call-poly "Enqueue Message.vi"("Message"="Exit", "Message Queue"=w440) -> ("error out"=w439:errorcluster)  [unwired: 8 in, 1 out]
      }
      event User Event {
        n184 = event-data() -> ("User Event"=w443:string, "Event Data"=w442:variant)  [unwired: 1 in]
        n185 = case shown="\"Exit EHL\"" w443 {
          tunnel: w442 -> [_ w445]
          tunnel: [_ w444] -> w441
          frame Default {
          }
          frame "Exit EHL" {
            # "#evangelio Termina\nla ejecucion del EHL"
            n186 = Variant To Data(type=TRUE, Variant=w445) -> (data=w444:bool)  [unwired: 1 in, 1 out]
          }
        }
      }
      event Panel Close? {
        w447 = TRUE
        n187 = event-data() -> ()  [unwired: 1 in, 1 out]
        n188 = call-poly "Enqueue Message.vi"("Priority Message? (F)"=w447, "Message"="Confirmar Salida", "Message Queue"=w448) -> ()  [unwired: 7 in, 2 out]
        n189 = event-data("Discard?"=w447) -> ()  [unwired: 1 in, 1 out]
      }
      event "generar1": Value Change {
        n190 = event-data() -> ("NewVal"=w453:bool)  [unwired: 1 in]
        n191 = Select(t="iniciarGEN_1", s=w453, f="detenerGEN") -> (s? t:f=w450:string)
        n192 = call-poly "Enqueue Message.vi"("Message"=w450, "Message Queue"=w454) -> ("error out"=w455:errorcluster)  [unwired: 8 in, 1 out]
      }
      event "genera2": Value Change {
        n193 = event-data() -> ()  [unwired: 1 in, 1 out]
        n194 = call-poly "Enqueue Message.vi"("Message"="iniciarGEN_burst", "Message Queue"=w460) -> ("error out"=w457:errorcluster)  [unwired: 8 in, 1 out]
        n195 = property on="TablaTempotal" class="Tbl (strict)"(error in=w457, "DisabledEnum"=T6."Enabled" ("Disabled")) -> (error out=w456:errorcluster)  [unwired: 1 in, 1 out]
      }
      event "seguir": Value Change {
        (unwired) T8 {"Estados"=enum."nivelMaxRef", "Data"=variant} ("MessageP08")
        n196 = event-data() -> ()  [unwired: 1 in, 1 out]
        n197 = call-poly "Enqueue Message.vi"("Message"="nivelMaxRef", "Message Queue"=w465) -> ("error out"=w463:errorcluster)  [unwired: 8 in, 1 out]
        n198 = property on="Tab" class="TabCtl (strict)"(error in=w463, "Value"=enum32{"Page 1", "Page 2"}."Page 2" ("Tab")) -> (error out=w462:errorcluster)  [unwired: 1 in, 1 out]
      }
      event "guardarParamLEQ": Value Change {
        (unwired) T8 {"Estados"=enum."nivelMaxRef", "Data"=variant} ("MessageP08")
        n199 = event-data() -> ()  [unwired: 1 in, 1 out]
        n200 = call-poly "Enqueue Message.vi"("Message"="nivelMaxRef", "Message Queue"=w467) -> ("error out"=w468:errorcluster)  [unwired: 8 in, 1 out]
      }
      event Value Change {
        (unwired) T8 {"Estados"=enum."FrecAmp1", "Data"=variant} ("MessageP08")
        n201 = event-data() -> ()  [unwired: 1 in, 1 out]
        n202 = Divide(x="AjusteAmp", y=T1 1000.0) -> (x/y=w469:T1)
        n203 = call-poly "Enqueue Message.vi"("Message Data"=w469, "Message"="EnviarVoltajeGEN", "Message Queue"=w473) -> ("error out"=w474:errorcluster)  [unwired: 7 in, 1 out]
      }
      event "guardar_Vref": Value Change {
        (unwired) T8 {"Estados"=enum."guardaVref", "Data"=variant} ("MessageP08")
        n204 = event-data() -> ()  [unwired: 1 in, 1 out]
        n205 = call-poly "Enqueue Message.vi"("Message"="guardaVref", "Message Queue"=w479) -> ("error out"=w477:errorcluster)  [unwired: 8 in, 1 out]
        n206 = property on="seguir" class="Bool"(error in=w477, "DisabledEnum"=T6."Enabled" ("Disabled")) -> (error out=w476:errorcluster)  [unwired: 1 in, 1 out]
      }
      event "TablaTempotal": Value Change {
        n207 = event-data() -> ("NewVal"=w481:string[][])  [unwired: 1 in]
        n208 = call-poly "Enqueue Message.vi"("Message Data"=w481, "Message"="llenaTablaTemporal", "Message Queue"=w483) -> ("error out"=w482:errorcluster)  [unwired: 7 in, 1 out]
      }
      event "cb_ponderacionTemp": Value Change {
        n209 = event-data() -> ("NewVal"=w485:string)  [unwired: 1 in]
        n210 = call-poly "Enqueue Message.vi"("Message Data"=w485, "Message"="TipoPonderacionTemporal", "Message Queue"=w487) -> ("error out"=w484:errorcluster)  [unwired: 7 in, 1 out]
      }
    }
    n211 = call "Error Handler - Event Handling Loop.vi"("error in (no error)"=w434, "Message Queue"=w431) -> ("dup error in"=w433:errorcluster, "Error?"=w432:bool)  [unwired: 7 in, 1 out]
    n212 = Or(x=w435, y=w432) -> (x .or. y?=w437:bool)
  }
  n213 = call "Inst_CNT90.vi"("All Message Queues in"=w1, "Prueba31 in"=w2) -> ()  [unwired: 9 in, 1 out]
  n214 = call "Inst_DS360.vi"("All Message Queues in"=w1, "Prueba08 in"=w2) -> ()  [unwired: 9 in, 1 out]
  n215 = call "Inst_K2002.vi"("All Message Queues in"=w1, "Prueba31 in"=w2) -> ()  [unwired: 9 in, 1 out]
  n216 = Merge Errors(w18, w17) -> (→"error out":errorcluster)
